vi "Get 2D CXT.vi"(7 "key description":string, 8 "sections":string[](array[string]), 9 "numeric":cxt[][](array[numeric]), 11 "info data":string) -> (0 "sections out":string[](array[string]), 1 "key found?":bool, 2 "value":cxt[][](array[numeric]) format="%.2f", 3 "info data out":string)   [LabVIEW 2020, in "infolib.lvlib"]
doc: "Reads matrix of CXT values. If section is entered it searches the key in the section(s).\nInput 'numeric' can be used to set default value.\nIf key is not found, the output value is equal to 'numeric' input.\nIf key is found, and element of matrix cannot be converted into data type, the default value of output matrix element is based on:\n- first element of 'numeric' input if available\n- otherwise NaN + NaN*i is used."
uses:
  infolib.lvlib
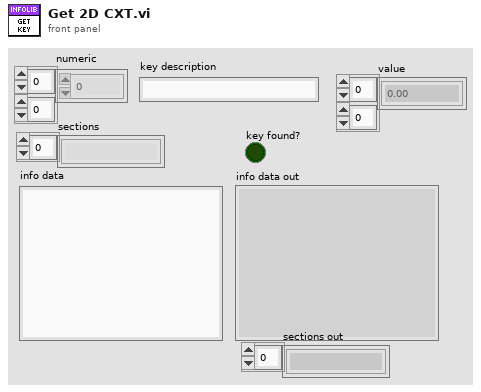
[diagram p1: front panel]
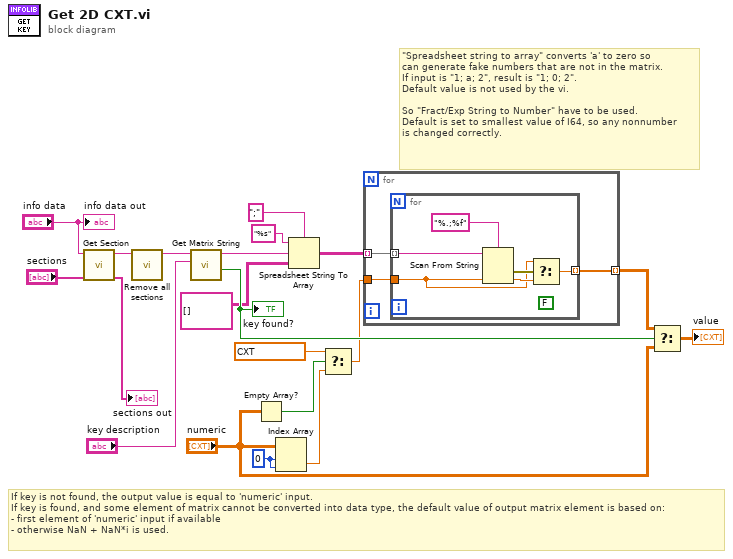
[diagram p0: block diagram]
diagram:
  w6 = 0 ("index (row)")
  # "If key is not found, the output value is equal to 'numeric' input.\nIf key is found, and some element of matrix cannot be converted into data type, the default value of output matrix element is based on:\n- first element of 'numeric' input if available\n- otherwise NaN + NaN*i is used."
  # "\"Spreadsheet string to array\" converts 'a' to zero so\ncan generate fake numbers that are not in the matrix.\nIf input is \"1; a; 2\", result is \"1; 0; 2\".\nDefault value is not used by the vi.\n\nSo \"Fract/Exp String to Number\" have to be used.\nDefault is set to smallest value of I64, so any nonnumber\nis changed correctly."
  n1 = call "Get Section.vi"("sections"="sections", "info data"="info data") -> ("sections out"=→"sections out":string[], "section part"=w20:string)  [unwired: 7 in, 1 out]
  n2 = call "Remove all sections.vi"("info data"=w20) -> ("info data out"=w18:string)  [unwired: 10 in]
  n3 = call "Get Matrix String.vi"("matrix key"="key description", "info data"=w18) -> ("key found?"=w11:bool, "matrix part"=w16:string)  [unwired: 8 in]
  "key found?" <- w11
  n4 = Empty Array?(array="numeric") -> (empty?=w4:bool)
  n5 = Index Array(array="numeric", index (row)=w6, index (col)=w6) -> (element=w5:cxt)
  n6 = Spreadsheet String To Array(delimiter (Tab)=";", format string="%s" ("format string (%_20f)"), spreadsheet string=w16, array type (2D Dbl)=string[][] [] ("v")) -> (array=w8:string[][])
  n7 = Select(t=cxt nan+nani ("x + iy"), s=w4, f=w5) -> (s? t:f=w1:cxt)
  n8 = for {
    tunnel: w8 -> [w23] mode=indexing
    tunnel: [w22] -> w7 mode=indexing
    tunnel: w1 -> [w21]
    n9 = for {
      tunnel: w23 -> [w28] mode=indexing
      tunnel: [w26] -> w22 mode=indexing
      tunnel: w21 -> [w24]
      (unwired) FALSE ("use system decimal point (T)")
      n10 = Scan From String(format string="%.;%f", input string=w28, default 1=w24) -> (error out=w27:errorcluster, output 1=w25:cxt)  [unwired: 2 in, 2 out]
      n11 = Select(t=w24, s=w27, f=w25) -> (s? t:f=w26:cxt)
    }
  }
  n12 = Select(t=w7, s=w11, f="numeric") -> (s? t:f=→"value":cxt[][])
  "info data out" <- "info data"
